vi "3.- Prueba 2 con GPIB.vi"() -> ()   [LabVIEW 2019]
uses:
  Controles/Amp_Frec.ctl
  <vilib>/Utility/error.llb/DialogType.ctl
  QMH_Support/Enqueue Message (Single).vi
  <vilib>/Utility/error.llb/Error Cluster From Error Code.vi
  <vilib>/ErrorRing/Error Ring.xnode
  QMH_Support/Message Queue.lvlib
  QMH_Support/User Event - Stop/User Event - Stop.lvlib
  DS360_GPIB/DS360_GPIB.lvlib
  K2202_GPIB/K2002_GPIB.lvlib
  CNT90_GPIB/CNT90_GPIB.lvlib
panel:
  out "mouse up?":bool
  out "EHL":i32
  out "# elements in queue":i32
  out "MHL":i32
  out "Instrumentos":i32
  in  "go_A":bool
  out "Voltaje a generar":dbl(knob) scale=0.0..10.0
  out "error out":errorcluster
  in  "stop":bool
  in  "generar":bool
  in  "Voltaje a Generar":dbl(slide)=7.0649350649350655 scale=0.0..10.0
  out "voltMon":dbl format="%.2f"
  out "frecMon":dbl format="%.2f"
  # "Ensayo Eléctrico Ponderación A"
  # "Monitoreo"
  # "Frecuencia"
  # "Hz"
  # "Voltaje"
  # "mV"
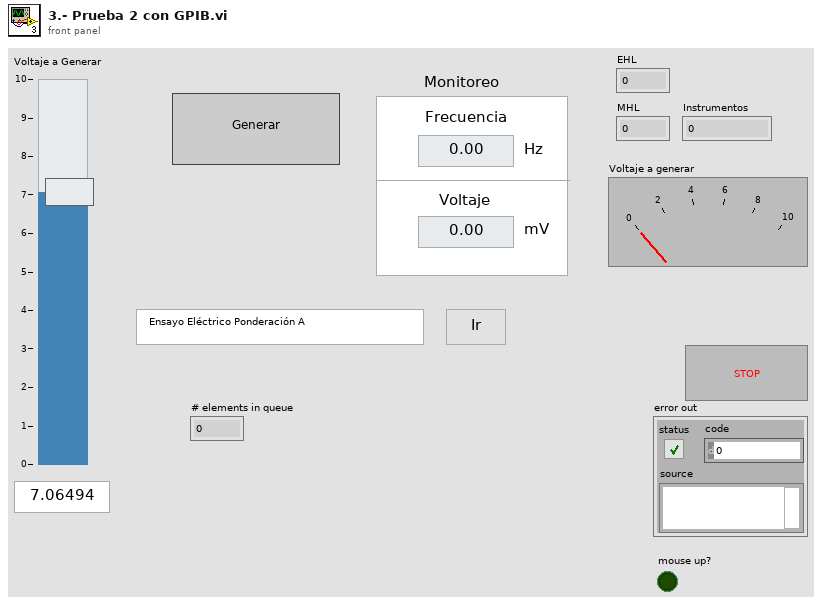
[diagram p1: front panel]
types:
  T1 = typedef "Message Queue.lvlib/All Message Queues.ctl" = cluster{"MHL":refnum<queue>, "DS360":refnum<queue>, "K2002":refnum<queue>, "CNT90":refnum<queue>, "Instrumentos":refnum<queue>}
  T2 = typedef "Amp_Frec.ctl" = cluster{"Ampl":dbl, "Frec":dbl}
  T3 = typedef "DialogType.ctl" = u16
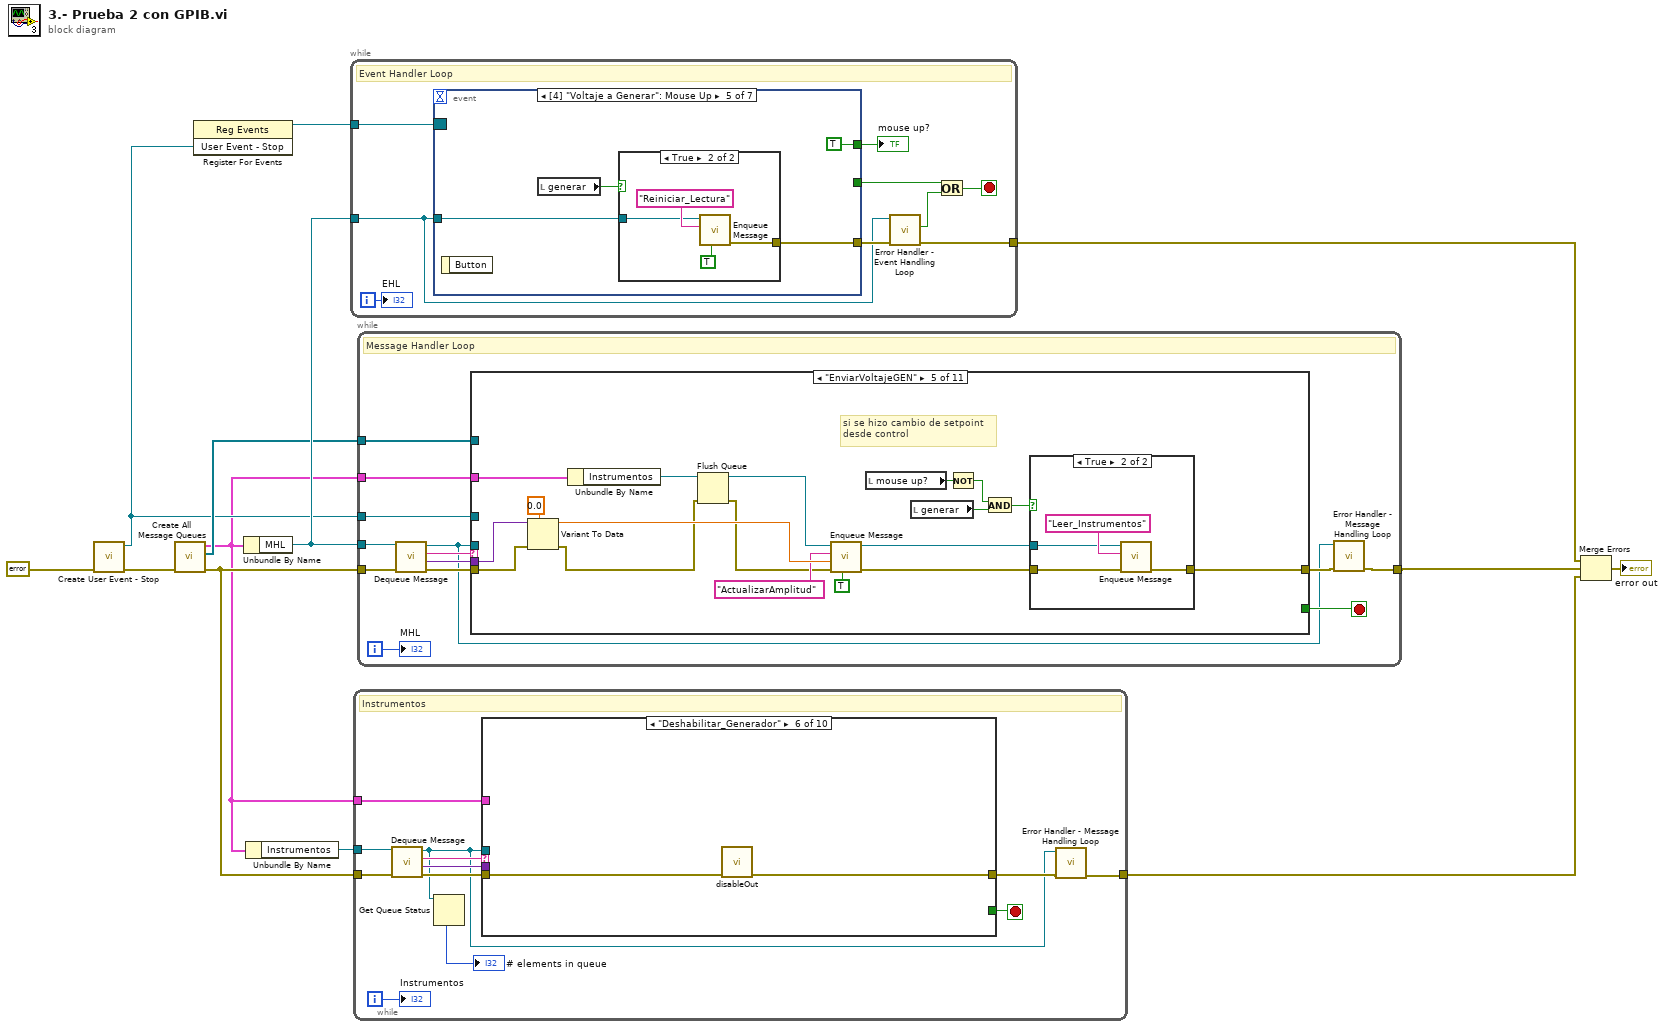
[diagram p0: block diagram]
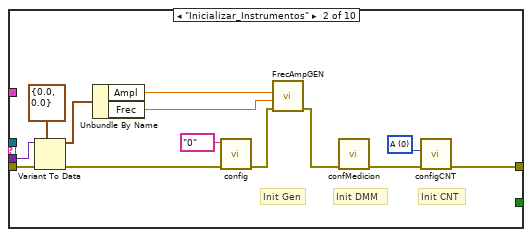
[diagram p3: hidden frame]
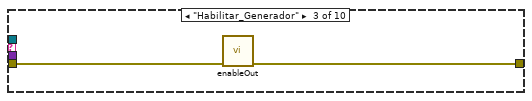
[diagram p4: hidden frame]
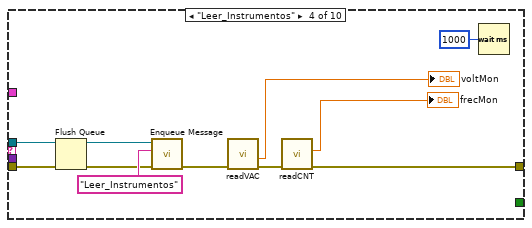
[diagram p5: hidden frame]
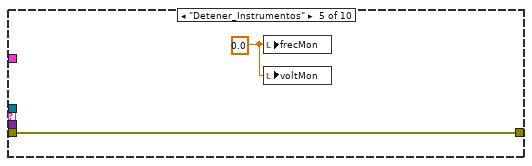
[diagram p6: hidden frame]
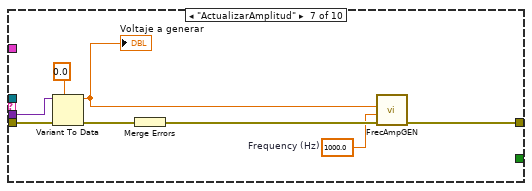
[diagram p7: hidden frame]
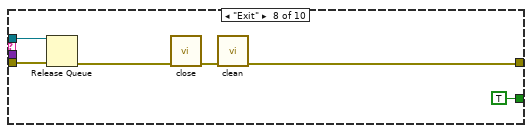
[diagram p8: hidden frame]
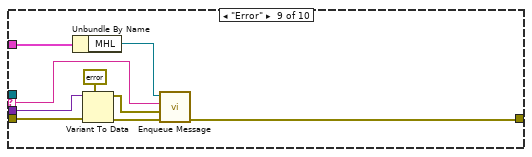
[diagram p9: hidden frame]
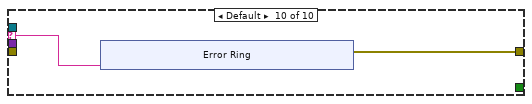
[diagram p10: hidden frame]
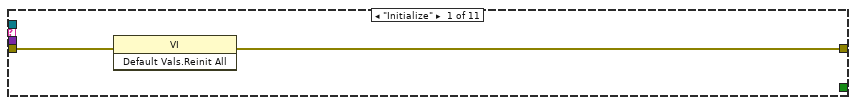
[diagram p11: hidden frame]
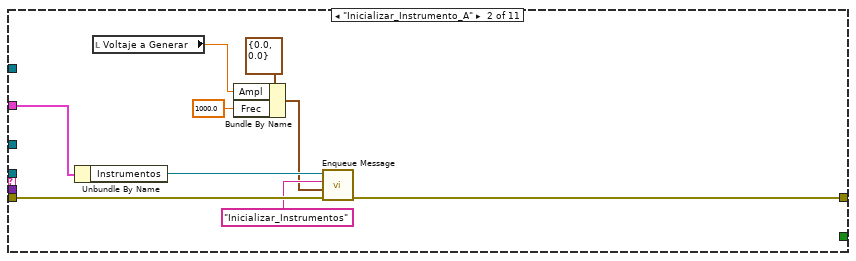
[diagram p12: hidden frame]
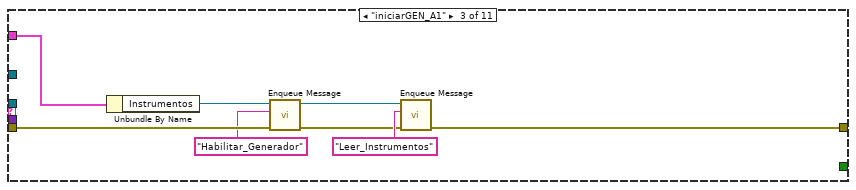
[diagram p13: hidden frame]
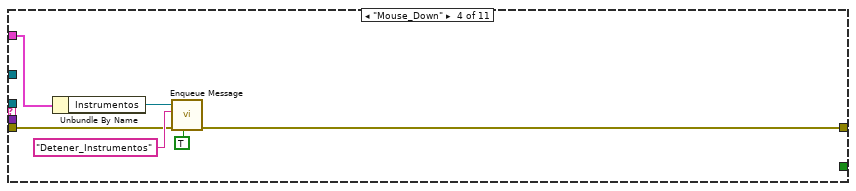
[diagram p14: hidden frame]
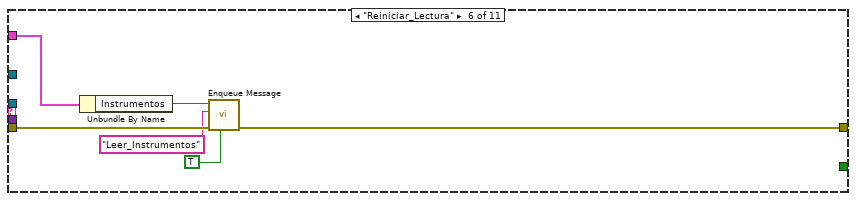
[diagram p16: hidden frame]
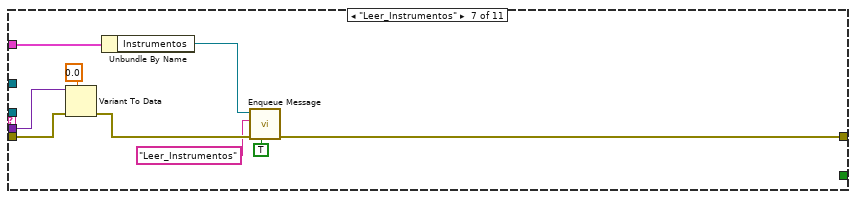
[diagram p17: hidden frame]
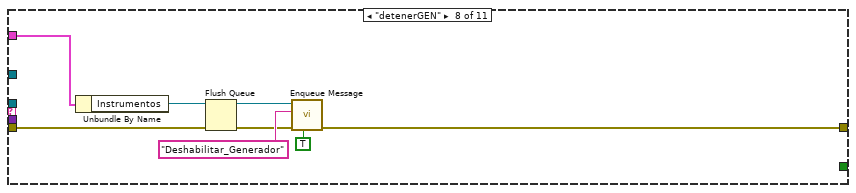
[diagram p18: hidden frame]
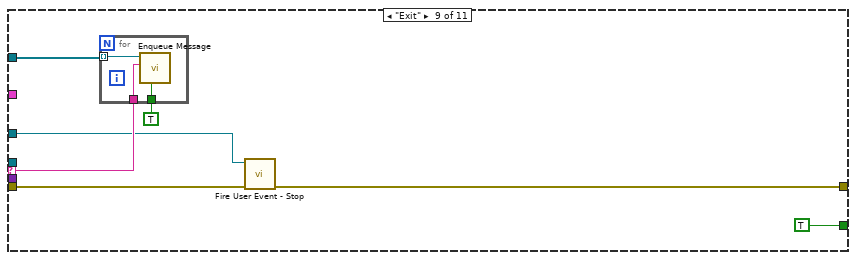
[diagram p19: hidden frame]
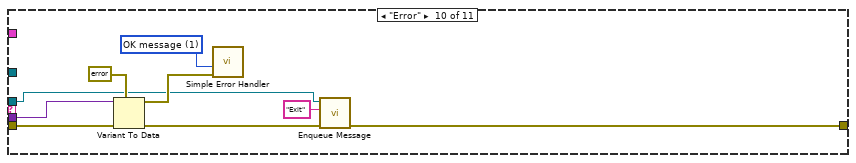
[diagram p20: hidden frame]
diagram:
  n1 = call "Create User Event - Stop.vi"("error in (no error)"=errorcluster {"status"=FALSE, "code"=0, "source"=""}) -> ("error out"=w7:errorcluster, "User Event - Stop"=w6:refnum<user-event>)  [unwired: 9 in]
  n2 = call "Create All Message Queues.vi"("error in (no error)"=w7) -> ("error out"=w3:errorcluster, "Queues Array"=w9:refnum<queue>[], "Message Queues out"=w1:T1)  [unwired: 8 in]
  n3 = register-events(w6) -> (reference out=w5:refnum<event-registration>)  [unwired: 2 in, 1 out]
  n4 = Unbundle By Name(w1) -> ("MHL"=w13:refnum<queue>)
  n5 = Unbundle By Name(w1) -> ("Instrumentos"=w4:refnum<queue>)
  n6 = while {
    tunnel: w13 -> [w19]
    tunnel: [w20] -> w12
    tunnel: w5 -> [w22]
    i -> [w15]
    stop <- w16 stop-if-true
    # "Event Handler Loop"
    n7 = event shown="[4] \"Voltaje a Generar\": Mouse Up" {
      selector: w22 -> [_ _ _ _ _ _ _]
      dyn-events: _ -> [_ _ _ _ _ _ _]
      timeout: _ -> [_ _ _ _ _ _ _]
      tunnel: w19 -> [w24 w27 w36 w42 w47 w56 _]
      tunnel: [w23 w26 w37 w41 w48 w54 _] -> w21
      tunnel: [_ _ _ _ _ _ TRUE] -> w18
      tunnel: [_ _ _ _ TRUE ("mouse up?") _ _] -> w14
      event "go_A": Value Change {
        n8 = event-data() -> ()  [unwired: 1 in, 1 out]
        n9 = call-poly "Enqueue Message.vi"("Message"="Inicializar_Instrumento_A" ("message"), "Message Queue"=w24) -> ("error out"=w23:errorcluster)  [unwired: 8 in, 1 out]
      }
      event "generar": Value Change {
        n10 = event-data() -> ("NewVal"=w28:bool)  [unwired: 1 in]
        n11 = Flush Queue(queue=w27) -> (queue out=w29:refnum<queue>, error out=w30:errorcluster)  [unwired: 1 in, 1 out]
        n12 = Select(t="iniciarGEN_A1" ("message"), s=w28, f="detenerGEN" ("message")) -> (s? t:f=w33:string)
        n13 = call-poly "Enqueue Message.vi"("Priority Message? (F)"=TRUE, "error in (no error)"=w30, "Message Data"="A1" ("message"), "Message"=w33, "Message Queue"=w29) -> ("error out"=w26:errorcluster)  [unwired: 5 in, 1 out]
      }
      event "Voltaje a Generar": Mouse Down {
        n14 = event-data() -> ()  [unwired: 1 in, 1 out]
        n15 = call-poly "Enqueue Message.vi"("Priority Message? (F)"=TRUE, "Message"="Mouse_Down" ("message"), "Message Queue"=w36) -> ("error out"=w37:errorcluster)  [unwired: 7 in, 1 out]
      }
      event "Voltaje a Generar": Value Change {
        n16 = event-data() -> ("NewVal"=w40:dbl)  [unwired: 1 in]
        n17 = call-poly "Enqueue Message.vi"("Priority Message? (F)"=TRUE, "Message Data"=w40, "Message"="EnviarVoltajeGEN" ("message"), "Message Queue"=w42) -> ("error out"=w41:errorcluster)  [unwired: 6 in, 1 out]
      }
      event "Voltaje a Generar": Mouse Up {
        n18 = event-data() -> ()  [unwired: 1 in, 1 out]
        n19 = local read "generar"() -> (w46:bool)
        n20 = case shown="True" w46 {
          tunnel: w47 -> [_ w51]
          tunnel: [errorcluster {"status"=FALSE, "code"=0, "source"=""} ("error out") w50] -> w48
          frame False {
          }
          frame True {
            n21 = call-poly "Enqueue Message.vi"("Priority Message? (F)"=TRUE, "Message"="Reiniciar_Lectura" ("message"), "Message Queue"=w51) -> ("error out"=w50:errorcluster)  [unwired: 7 in, 1 out]
          }
        }
      }
      event "stop": Value Change {
        n22 = event-data() -> ()  [unwired: 1 in, 1 out]
        n23 = call-poly "Enqueue Message.vi"("Message"="Exit", "Message Queue"=w56) -> ("error out"=w54:errorcluster)  [unwired: 8 in, 1 out]
      }
      event User Event {
        n24 = event-data() -> ()  [unwired: 1 in, 1 out]
      }
    }
    "mouse up?" <- w14
    n25 = call "Error Handler - Event Handling Loop.vi"("error in (no error)"=w21, "Message Queue"=w19) -> ("dup error in"=w20:errorcluster, "Error?"=w17:bool)  [unwired: 7 in, 1 out]
    n26 = Or(x=w18, y=w17) -> (x .or. y?=w16:bool)
    "EHL" <- w15
  }
  n27 = while {
    tunnel: w4 -> [w69]
    tunnel: w3 -> [w68]
    tunnel: [w61] -> w2
    tunnel: w1 -> [w60]
    i -> [w63]
    stop <- w64 stop-if-true
    # "Instrumentos"
    n28 = call "Dequeue Message.vi"("error in (no error)"=w68, "Message Queue"=w69) -> ("error out"=w67:errorcluster, "Message Data"=w65:variant, "Message"=w66:string, "dup Message Queue"=w59:refnum<queue>)  [unwired: 6 in]
    n29 = Get Queue Status(queue=w59) -> (# elements in queue=→"# elements in queue":i32)  [unwired: 2 in, 7 out]
    n30 = case shown="\"Deshabilitar_Generador\"" w66 {
      selector: w66 -> [_ _ _ _ _ _ _ _ w118 w125]
      tunnel: w67 -> [w70 w83 w85 w94 w98 w100 w103 w114 w120 _]
      tunnel: w65 -> [_ w81 _ _ _ _ w107 _ w119 _]
      tunnel: w59 -> [_ _ _ w88 _ _ _ w113 _ _]
      tunnel: [w70 w76 w84 w93 w98 w99 w105 w110 w117 w124] -> w62
      tunnel: [_ _ _ _ _ _ _ TRUE _ _] -> w64
      tunnel: w60 -> [_ _ _ _ _ _ _ _ w116 _]
      frame "Initialize" {
      }
      frame "Inicializar_Instrumentos" {
        w73 = 0 items=["A", "B"] ("Channel  1")
        # "Init CNT"
        # "Init DMM"
        # "Init Gen"
        n31 = Variant To Data(error in=w83, type=T2 {"Ampl"=0.0, "Frec"=0.0}, Variant=w81) -> (data=w80:T2, error out=w79:errorcluster)
        n32 = Unbundle By Name(w80) -> ("Ampl"=w78:dbl, "Frec"=w77:dbl)
        n33 = call "config.vi"("error in (no error)"=w79, "Impedancia"="0") -> ("error out"=w74:errorcluster)  [unwired: 9 in]
        n34 = call "FrecAmpGEN.vi"("error in (no error)"=w74, "Frec (Hz)"=w77, "Amplitud (Vrms)"=w78) -> ("error out"=w72:errorcluster)  [unwired: 8 in]
        n35 = call "confMedicion.vi"("error in (no error)"=w72) -> ("error out"=w71:errorcluster)  [unwired: 10 in]
        n36 = call "configCNT.vi"("error in (no error)"=w71, "Channel  1"=w73) -> ("error out"=w76:errorcluster)  [unwired: 9 in]
      }
      frame "Habilitar_Generador" {
        n37 = call "enableOut.vi"("error in (no error)"=w85) -> ("error out"=w84:errorcluster)  [unwired: 10 in]
      }
      frame "Leer_Instrumentos" {
        n38 = Flush Queue(queue=w88, error in (no error)=w94) -> (queue out=w87:refnum<queue>, error out=w89:errorcluster)  [unwired: 1 out]
        n39 = call-poly "Enqueue Message.vi"("error in (no error)"=w89, "Message"="Leer_Instrumentos", "Message Queue"=w87) -> ("error out"=w95:errorcluster)  [unwired: 7 in, 1 out]
        n40 = call "readVAC.vi"("error in (no error)"=w95) -> ("error out"=w86:errorcluster, "medicion"=→"voltMon":dbl)  [unwired: 8 in, 1 out]
        n41 = call "readCNT.vi"("error in (no error)"=w86) -> ("error out"=w93:errorcluster, "medicion"=→"frecMon":dbl)  [unwired: 9 in]
        n42 = Wait (ms)(milliseconds to wait=u32 1000) -> ()  [unwired: 1 out]
      }
      frame "Detener_Instrumentos" {
        w97 = 0.0 ("frecMon")
        n43 = local write "frecMon"(w97) -> ()
        n44 = local write "voltMon"(w97) -> ()
      }
      frame "Deshabilitar_Generador" {
        n45 = call "disableOut.vi"("error in (no error)"=w100) -> ("error out"=w99:errorcluster)  [unwired: 10 in]
      }
      frame "ActualizarAmplitud" {
        w101 = 1000.0  # Frequency (Hz)
        n46 = Variant To Data(error in=w103, type=0.0, Variant=w107) -> (data=w104:dbl, error out=w106:errorcluster)
        "Voltaje a generar" <- w104
        n47 = Merge Errors(w106) -> (w102:errorcluster)
        n48 = call "FrecAmpGEN.vi"("error in (no error)"=w102, "Frec (Hz)"=w101, "Amplitud (Vrms)"=w104) -> ("error out"=w105:errorcluster)  [unwired: 8 in]
      }
      frame "Exit" {
        n49 = Release Queue(queue=w113, error in (no error)=w114) -> (error out=w111:errorcluster)  [unwired: 1 in, 2 out]
        n50 = call "close.vi"("error in (no error)"=w111) -> ("error out"=w109:errorcluster)  [unwired: 10 in]
        n51 = call "clean.vi"("error in (no error)"=w109) -> ("error out"=w110:errorcluster)  [unwired: 10 in]
      }
      frame "Error" {
        n52 = Unbundle By Name(w116) -> ("MHL"=w115:refnum<queue>)
        n53 = Variant To Data(error in=w120, type=errorcluster {"status"=FALSE, "code"=0, "source"=""} ("error constant"), Variant=w119) -> (data=w121:errorcluster, error out=w122:errorcluster)
        n54 = call-poly "Enqueue Message.vi"("error in (no error)"=w122, "Message Data"=w121, "Message"=w118, "Message Queue"=w115) -> ("error out"=w117:errorcluster)  [unwired: 6 in, 1 out]
      }
      frame Default {
        n55 = xnode "Error Ring"("parameter 0"=w125) -> ("error out"=w124:errorcluster)
      }
    }
    n56 = call "Error Handler - Message Handling Loop.vi"("error in (no error)"=w62, "Message Queue"=w59) -> ("dup error in"=w61:errorcluster)  [unwired: 8 in, 1 out]
    "Instrumentos" <- w63
  }
  n57 = while {
    tunnel: w13 -> [w145]
    tunnel: w3 -> [w144]
    tunnel: [w136] -> w11
    tunnel: w9 -> [w140]
    tunnel: w6 -> [w138]
    tunnel: w1 -> [w134]
    i -> [w133]
    stop <- w139 stop-if-true
    # "Message Handler Loop"
    n58 = call "Dequeue Message.vi"("error in (no error)"=w144, "Message Queue"=w145) -> ("error out"=w141:errorcluster, "Message Data"=w142:variant, "Message"=w143:string, "dup Message Queue"=w135:refnum<queue>)  [unwired: 6 in]
    n59 = case shown="\"EnviarVoltajeGEN\"" w143 {
      selector: w143 -> [_ _ _ _ _ _ _ _ w222 _ w237]
      tunnel: w142 -> [_ _ _ _ w186 _ w206 _ _ w227 _]
      tunnel: w141 -> [w147 w155 w164 w167 w187 w199 w207 w215 w219 w230 _]
      tunnel: w135 -> [_ _ _ _ _ _ _ _ _ w228 _]
      tunnel: [w146 w156 w158 w170 w176 w195 w203 w213 w218 w229 w236] -> w137
      tunnel: w140 -> [_ _ _ _ _ _ _ _ w223 _ _]
      tunnel: [_ _ _ _ _ _ _ _ TRUE _ _] -> w139
      tunnel: w138 -> [_ _ _ _ _ _ _ _ w217 _ _]
      tunnel: w134 -> [_ w153 w163 w166 w185 w198 w205 w214 _ _ _]
      frame "Initialize" {
        n60 = invoke class="VI" method="Default Vals.Reinit All"(error in=w147) -> (error out=w146:errorcluster)  [unwired: 2 in, 2 out]
      }
      frame "Inicializar_Instrumento_A" {
        n61 = Unbundle By Name(w153) -> ("Instrumentos"=w152:refnum<queue>)
        n62 = local read "Voltaje a Generar"() -> (w149:dbl)
        n63 = Bundle By Name(cluster=T2 {"Ampl"=0.0, "Frec"=0.0}, "Ampl"=w149, "Frec"=1000.0) -> (w150:T2)
        n64 = call-poly "Enqueue Message.vi"("error in (no error)"=w155, "Message Data"=w150, "Message"="Inicializar_Instrumentos", "Message Queue"=w152) -> ("error out"=w156:errorcluster)  [unwired: 6 in, 1 out]
      }
      frame "iniciarGEN_A1" {
        n65 = Unbundle By Name(w163) -> ("Instrumentos"=w162:refnum<queue>)
        n66 = call-poly "Enqueue Message.vi"("error in (no error)"=w164, "Message"="Habilitar_Generador", "Message Queue"=w162) -> ("error out"=w159:errorcluster, "dup Message Queue"=w157:refnum<queue>)  [unwired: 7 in]
        n67 = call-poly "Enqueue Message.vi"("error in (no error)"=w159, "Message"="Leer_Instrumentos", "Message Queue"=w157) -> ("error out"=w158:errorcluster)  [unwired: 7 in, 1 out]
      }
      frame "Mouse_Down" {
        n68 = Unbundle By Name(w166) -> ("Instrumentos"=w165:refnum<queue>)
        n69 = call-poly "Enqueue Message.vi"("Priority Message? (F)"=TRUE, "error in (no error)"=w167, "Message"="Detener_Instrumentos", "Message Queue"=w165) -> ("error out"=w170:errorcluster)  [unwired: 6 in, 1 out]
      }
      frame "EnviarVoltajeGEN" {
        # "si se hizo cambio de setpoint\ndesde control"
        n70 = Variant To Data(error in=w187, type=0.0, Variant=w186) -> (data=w183:dbl, error out=w179:errorcluster)
        n71 = Unbundle By Name(w185) -> ("Instrumentos"=w184:refnum<queue>)
        n72 = Flush Queue(queue=w184, error in (no error)=w179) -> (queue out=w180:refnum<queue>, error out=w178:errorcluster)  [unwired: 1 out]
        n73 = call-poly "Enqueue Message.vi"("Priority Message? (F)"=TRUE, "error in (no error)"=w178, "Message Data"=w183, "Message"="ActualizarAmplitud", "Message Queue"=w180) -> ("error out"=w177:errorcluster, "dup Message Queue"=w175:refnum<queue>)  [unwired: 5 in]
        n74 = local read "mouse up?"() -> (w172:bool)
        n75 = local read "generar"() -> (w174:bool)
        n76 = Not(x=w172) -> (.not. x?=w171:bool)
        n77 = And(x=w171, y=w174) -> (x .and. y?=w173:bool)
        n78 = case shown="True" w173 {
          tunnel: w177 -> [w189 w192]
          tunnel: [w189 w191] -> w176
          tunnel: w175 -> [_ w190]
          frame False {
          }
          frame True {
            n79 = call-poly "Enqueue Message.vi"("error in (no error)"=w192, "Message"="Leer_Instrumentos" ("message"), "Message Queue"=w190) -> ("error out"=w191:errorcluster)  [unwired: 7 in, 1 out]
          }
        }
      }
      frame "Reiniciar_Lectura" {
        n80 = Unbundle By Name(w198) -> ("Instrumentos"=w197:refnum<queue>)
        n81 = call-poly "Enqueue Message.vi"("Priority Message? (F)"=TRUE, "error in (no error)"=w199, "Message"="Leer_Instrumentos", "Message Queue"=w197) -> ("error out"=w195:errorcluster)  [unwired: 6 in, 1 out]
      }
      frame "Leer_Instrumentos" {
        n82 = Variant To Data(error in=w207, type=0.0, Variant=w206) -> (error out=w204:errorcluster)  [unwired: 1 out]
        n83 = Unbundle By Name(w205) -> ("Instrumentos"=w200:refnum<queue>)
        n84 = call-poly "Enqueue Message.vi"("Priority Message? (F)"=TRUE, "error in (no error)"=w204, "Message"="Leer_Instrumentos", "Message Queue"=w200) -> ("error out"=w203:errorcluster)  [unwired: 6 in, 1 out]
      }
      frame "detenerGEN" {
        n85 = Unbundle By Name(w214) -> ("Instrumentos"=w210:refnum<queue>)
        n86 = Flush Queue(queue=w210, error in (no error)=w215) -> (queue out=w209:refnum<queue>, error out=w211:errorcluster)  [unwired: 1 out]
        n87 = call-poly "Enqueue Message.vi"("Priority Message? (F)"=TRUE, "error in (no error)"=w211, "Message"="Deshabilitar_Generador", "Message Queue"=w209) -> ("error out"=w213:errorcluster)  [unwired: 6 in, 1 out]
      }
      frame "Exit" {
        n88 = for {
          tunnel: w223 -> [w226] mode=indexing
          tunnel: w222 -> [w225]
          tunnel: TRUE -> [w224]
          n89 = call-poly "Enqueue Message.vi"("Priority Message? (F)"=w224, "Message"=w225, "Message Queue"=w226) -> ()  [unwired: 7 in, 2 out]
        }
        n90 = call "Fire User Event - Stop.vi"("error in (no error)"=w219, "User Event - Stop"=w217) -> ("error out"=w218:errorcluster)  [unwired: 9 in]
      }
      frame "Error" {
        w234 = T3 1 items=["no dialog", "OK message", "continue or stop message", "OK message + warnings", "continue/stop + warnings"] ("type of dialog (OK msg:1)")
        n91 = Variant To Data(error in=w230, type=errorcluster {"status"=FALSE, "code"=0, "source"=""} ("error out"), Variant=w227) -> (data=w232:errorcluster, error out=w231:errorcluster)
        n92 = call <vilib>:"Simple Error Handler.vi"("type of dialog (OK msg:1)"=w234, "error in (no error)"=w232) -> ()  [unwired: 3 in, 5 out]
        n93 = call-poly "Enqueue Message.vi"("error in (no error)"=w231, "Message"="Exit", "Message Queue"=w228) -> ("error out"=w229:errorcluster)  [unwired: 7 in, 1 out]
      }
      frame Default {
        n94 = xnode "Error Ring"("parameter 0"=w237) -> ("error out"=w236:errorcluster)
      }
    }
    n95 = call "Error Handler - Message Handling Loop.vi"("error in (no error)"=w137, "Message Queue"=w135) -> ("dup error in"=w136:errorcluster)  [unwired: 8 in, 1 out]
    "MHL" <- w133
  }
  n96 = Merge Errors(w12, w11, w2) -> (→"error out":errorcluster)
